vi "test Get Port Number.vi"(8 "error in":errorcluster, 11 "TestCase in":refnum<class "Scripting.lvclass">) -> (0 "error out":errorcluster, 3 "TestCase out":refnum<class "Scripting.lvclass">)   [LabVIEW 2020, in "Scripting.lvclass"]
uses:
  Scripting.lvclass
  Scripting.lvclass/Scripting.ctl
  <vilib>/addons/_JKI Toolkits/VI Tester/TestCase.llb/TestCase.lvclass
  Scripting/Ballard ARINC 429 Scripting.lvlib
  Scripting/ARINC 429 Scripting.lvlib
  C:/Program Files (x86)/National Instruments/LabVIEW 2020/vi.lib/addons/_JKI Toolkits/VI Tester/TestCase.llb/TestCase.lvclass
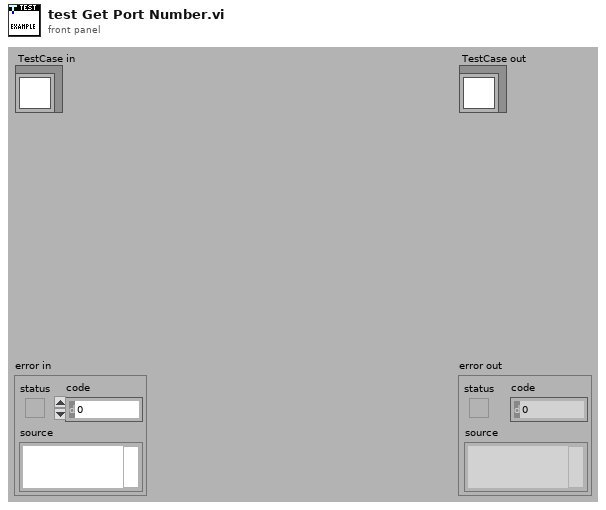
[diagram p1: front panel]
types:
  T1 = typedef "Custom Device API.lvlib/Custom Device Item Ref.ctl" = u64
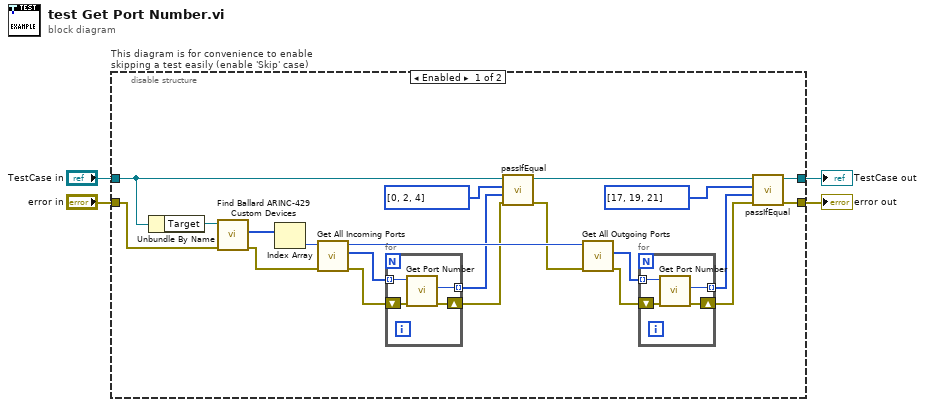
[diagram p0: block diagram]
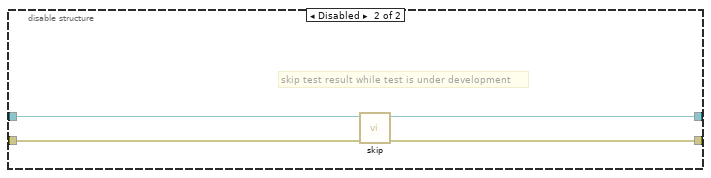
[diagram p2: hidden frame]
diagram:
  n1 = disable-structure "This diagram is for convenience to enable skipping a test easily (enable 'Skip' case)" shown="Enabled" {
    disable-tunnel: "TestCase in" -> [w23 w37]
    disable-tunnel: [w20 w35] -> w1
    disable-tunnel: [w6 w36] -> w3
    disable-tunnel: "error in" -> [w9 w34]
    frame Enabled {
      n2 = Unbundle By Name(w23) -> ("Target"=w25:refnum<k24>)
      n3 = call "Find Ballard ARINC-429 Custom Devices.vi"("error in"=w9, "target in"=w25) -> ("error out"=w22:errorcluster, "Ballard ARINC 429 custom devices"=w5:u64[])  [unwired: 7 in, 1 out]
      n4 = Index Array(array=w5) -> (element=w24:u64)  [unwired: 1 in]
      n5 = call "Get All Incoming Ports.vi"("error in"=w22, "Ballard ARINC 429 ref"=w24) -> ("error out"=w18:errorcluster, "Port refs"=w17:T1[], "Ballard ARINC 429 ref out"=w21:T1)  [unwired: 7 in]
      n6 = for {
        tunnel: w17 -> [w32] mode=indexing
        shift-right: [w31] -> w10
        shift-left: w18 -> [w33]
        tunnel: [w30] -> w16 mode=indexing
        n7 = call "Get Port Number.vi"("error in"=w33, "port ref in"=w32) -> ("error out"=w31:errorcluster, "port number"=w30:u16)  [unwired: 6 in, 2 out]
      }
      n8 = call-dynamic "passIfEqual.vi"("error in (no error)"=w10, "y"=w16, "x"=u16[] [0, 2, 4], "TestCase in"=w23) -> ("error out"=w8:errorcluster, "TestCase out"=w19:refnum<class "Scripting.lvclass">)  [unwired: 6 in]
      n9 = call "Get All Outgoing Ports.vi"("error in"=w8, "Ballard ARINC 429 ref"=w21) -> ("error out"=w11:errorcluster, "Port refs"=w14:T1[])  [unwired: 7 in, 1 out]
      n10 = for {
        shift-right: [w28] -> w7
        shift-left: w11 -> [w29]
        tunnel: [w27] -> w13 mode=indexing
        tunnel: w14 -> [w26] mode=indexing
        n11 = call "Get Port Number.vi"("error in"=w29, "port ref in"=w26) -> ("error out"=w28:errorcluster, "port number"=w27:u16)  [unwired: 6 in, 2 out]
      }
      n12 = call-dynamic "passIfEqual.vi"("error in (no error)"=w7, "y"=w13, "x"=u16[] [17, 19, 21], "TestCase in"=w19) -> ("error out"=w6:errorcluster, "TestCase out"=w20:refnum<class "Scripting.lvclass">)  [unwired: 6 in]
    }
    frame Disabled {
      # "skip test result while test is under development"
      n13 = call <vilib>:"skip.vi"("error in (no error)"=w34, "TestCase in"=w37) -> ("error out"=w36:errorcluster, "TestCase out"=w35:refnum<class "Scripting.lvclass">)  [unwired: 8 in]
    }
  }
  "error out" <- w3
  "TestCase out" <- w1
